vi "Generate Table.vi"() -> ()   [LabVIEW 2017]
panel:
  in  "Distance of Sensor Front to Back":dbl=34.0
  out "min time (in/sec)":dbl
  out "Feet/sec":dbl
  out "Distance":dbl
  out "Angle":dbl
  in  "Tape Width":dbl=2.0
  in  "Distance of Sensors Left to Right":dbl=20.0
  in  "Time between Rise of one to fall of other":dbl
  in  "Velocity(in/s":dbl=200.0
  out "Waveform Graph":waveform(dbl)(graph)
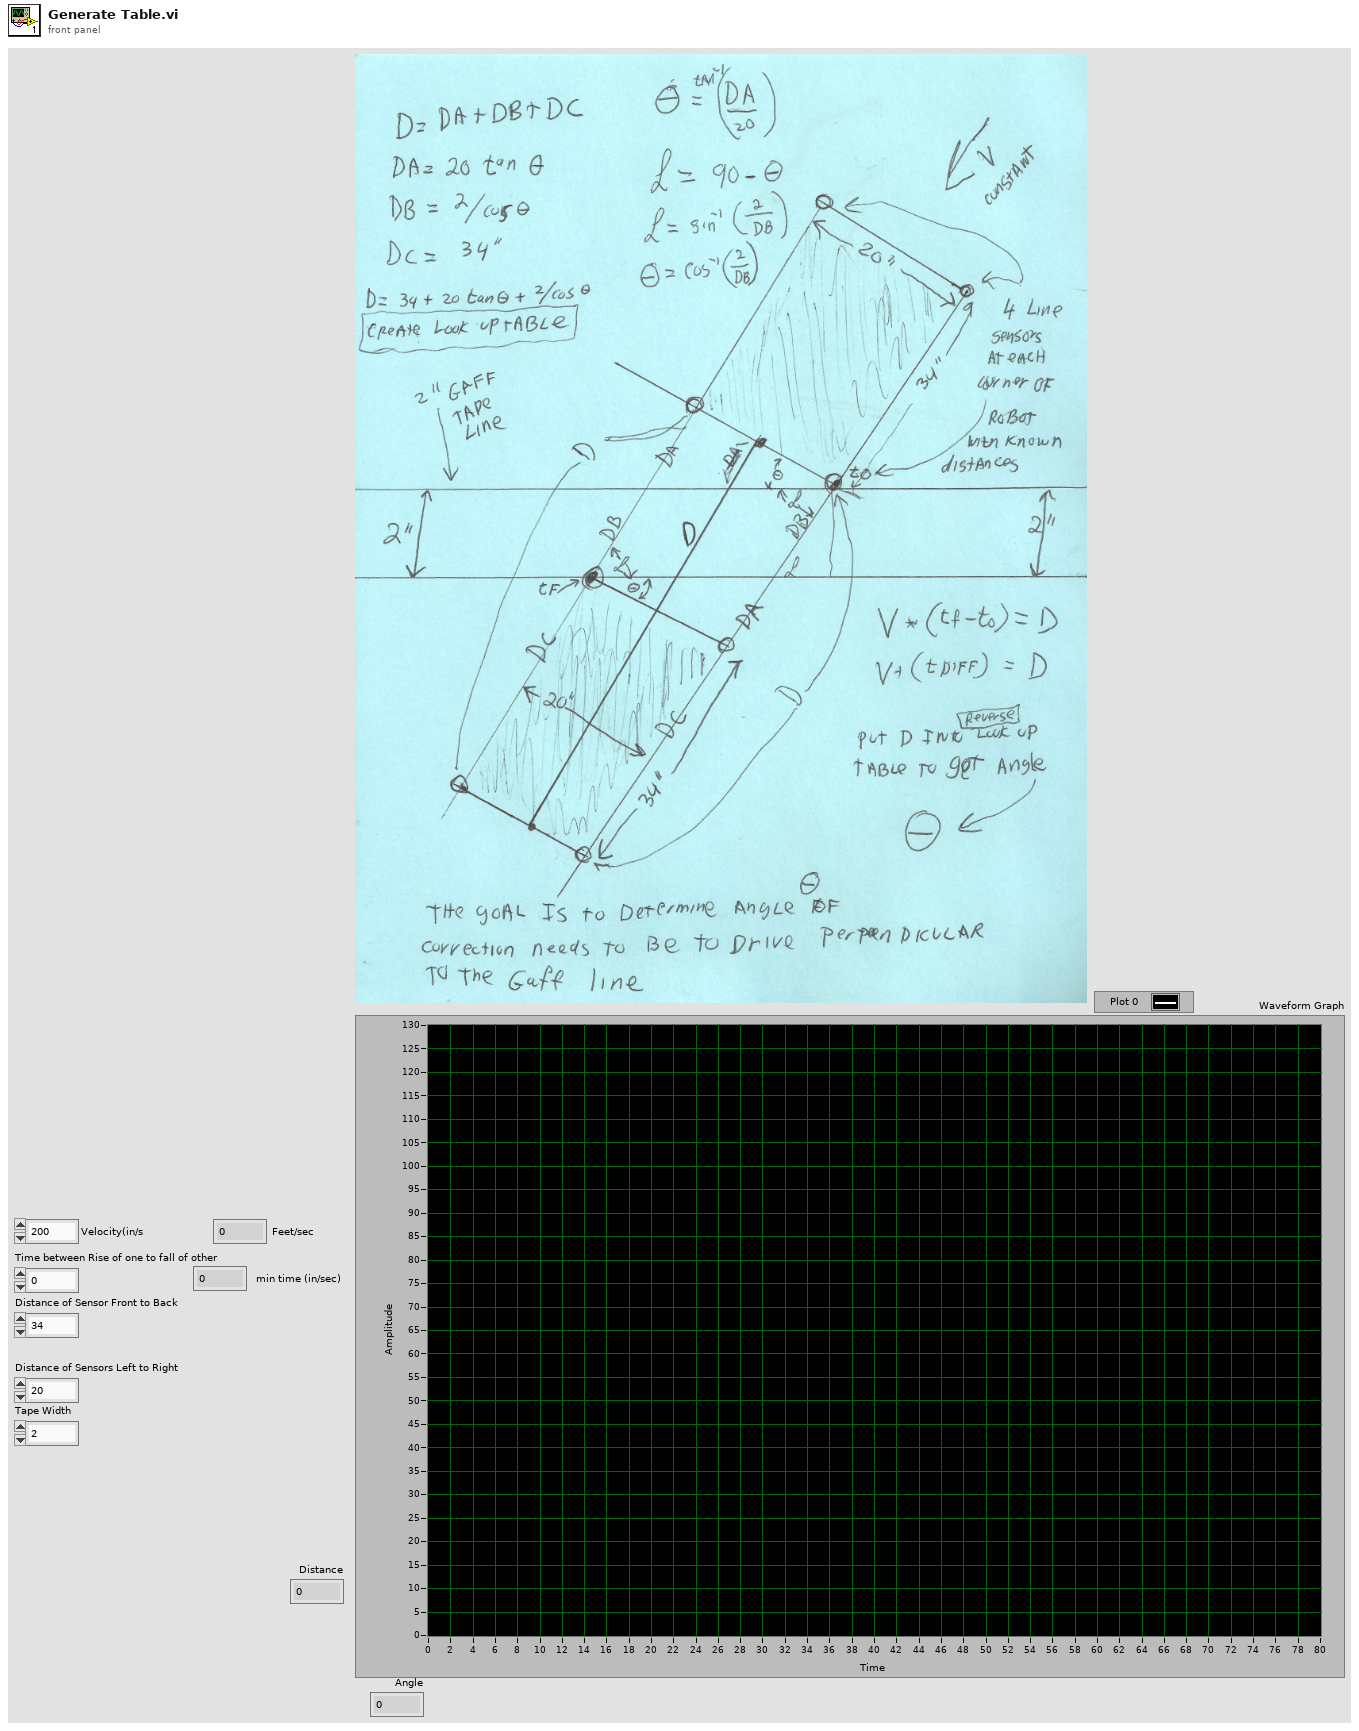
[diagram p1: front panel]
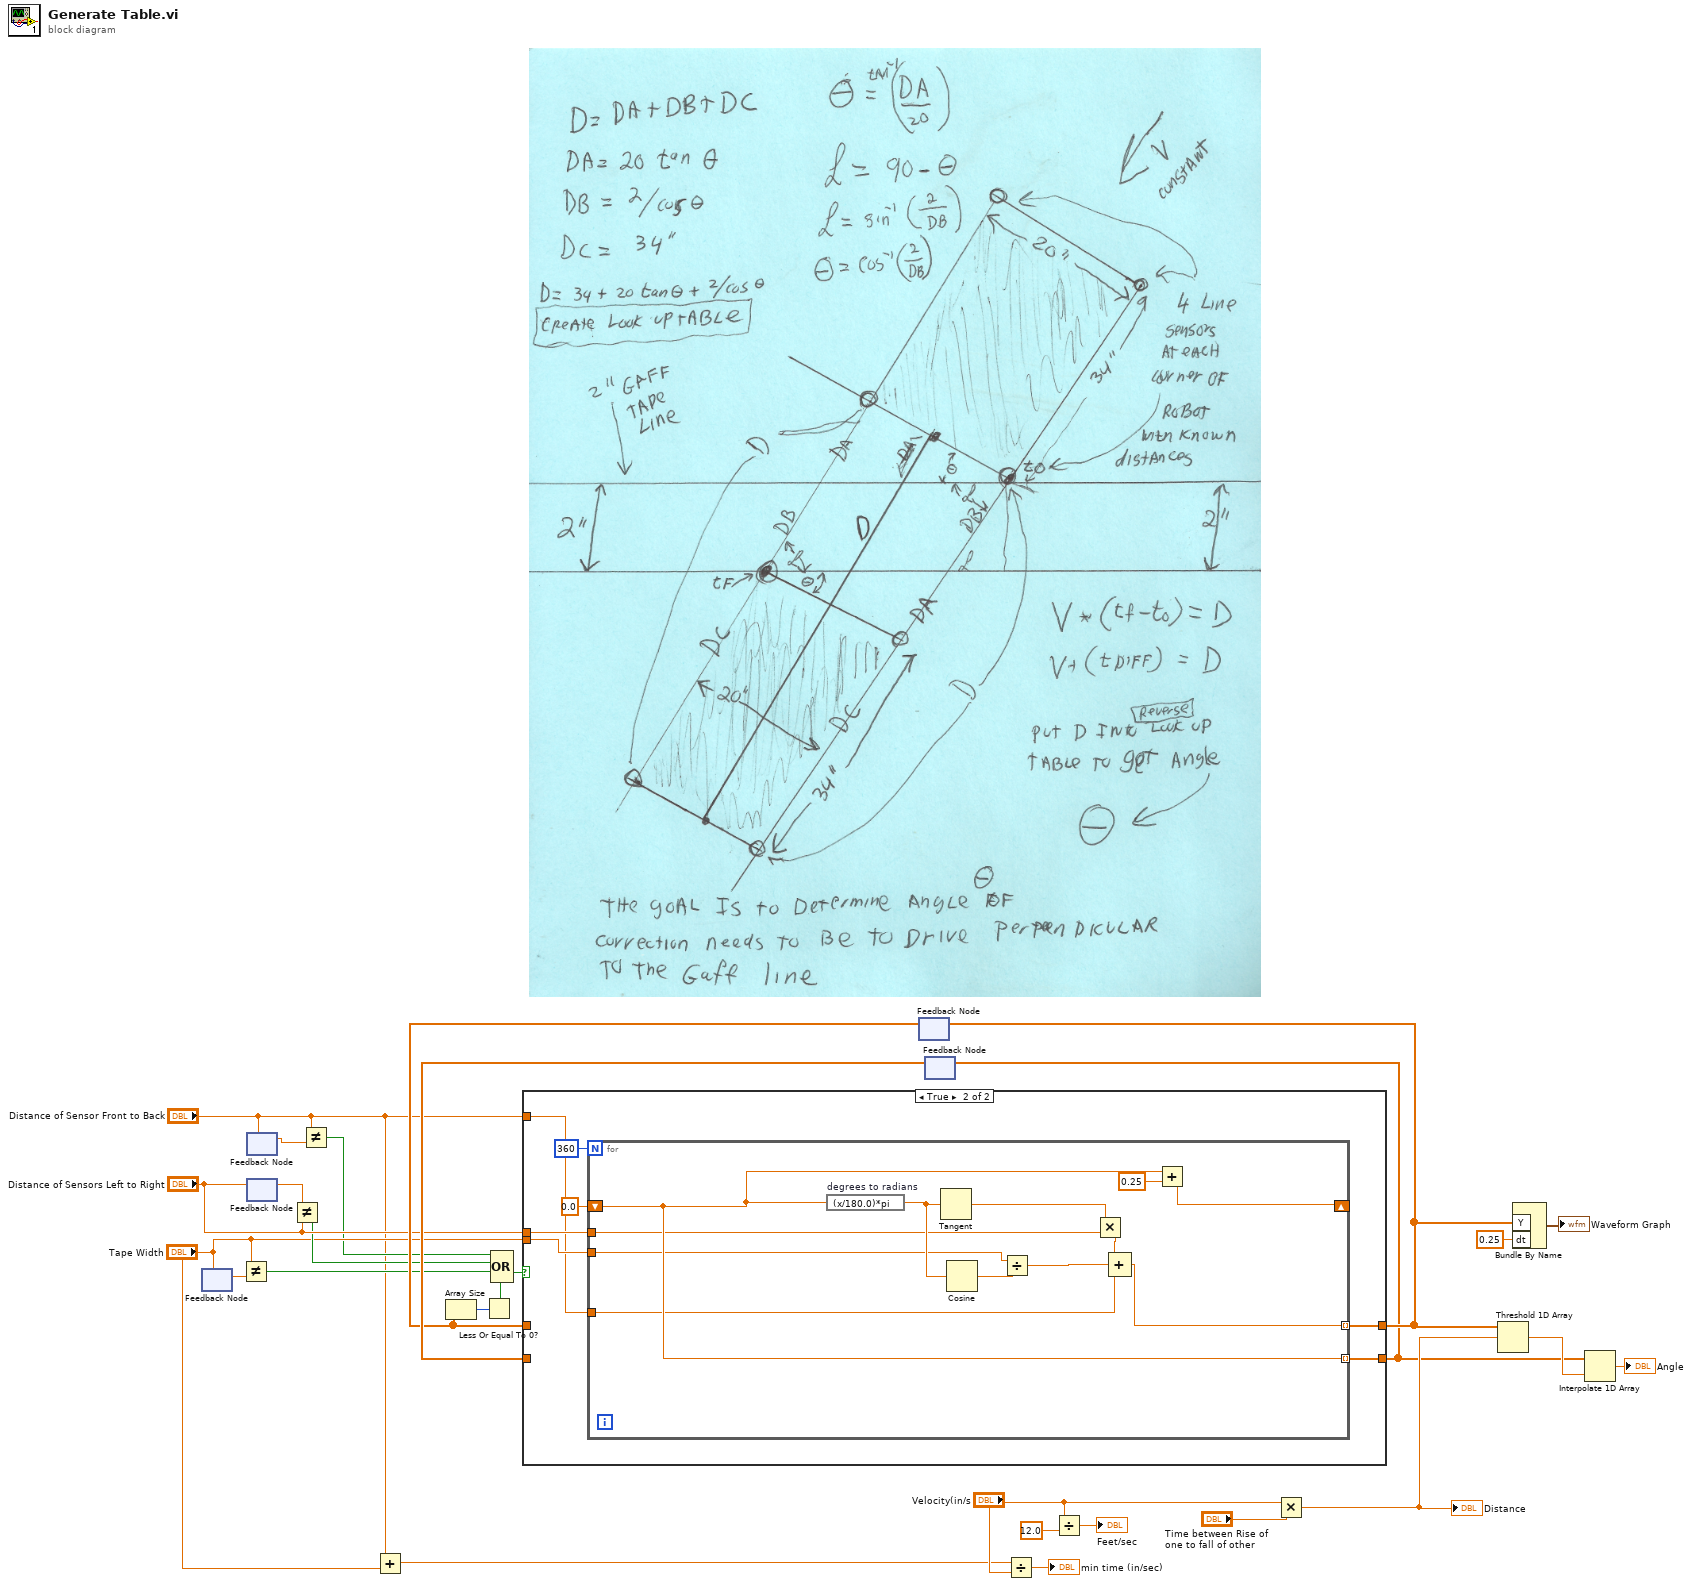
[diagram p0: block diagram]
diagram:
  n1 = feedback-in #1("Tape Width") -> ()
  n2 = feedback #1() -> (w14:dbl)  [unwired: 1 in]
  n3 = Not Equal?(x="Tape Width", y=w14) -> (x != y?=w13:bool)
  n4 = feedback #2() -> (w4:dbl)  [unwired: 1 in]
  n5 = feedback-in #2("Distance of Sensor Front to Back") -> ()
  n6 = feedback #3() -> (w11:dbl)  [unwired: 1 in]
  n7 = feedback-in #3("Distance of Sensors Left to Right") -> ()
  n8 = Not Equal?(x=w11, y="Distance of Sensors Left to Right") -> (x != y?=w10:bool)
  n9 = Not Equal?(x="Distance of Sensor Front to Back", y=w4) -> (x != y?=w3:bool)
  n10 = Add(x="Distance of Sensor Front to Back", y="Tape Width") -> (x+y=w2:dbl)
  n11 = feedback #4() -> (w18:dbl[])  [unwired: 1 in]
  n12 = Array Size(array=w18) -> (size(s)=w17:i32)
  n13 = Less Or Equal To 0?(x=w17) -> (x <= 0?=w16:bool)
  n14 = Compound Arithmetic op=OR(w3, w10, w13, w16) -> (w15:bool)
  n15 = feedback #5() -> (w19:dbl[])  [unwired: 1 in]
  n16 = case shown="True" w15 {
    tunnel: [w29 w35] -> w21
    tunnel: [w28 w34] -> w20
    tunnel: w18 -> [w29 _]
    tunnel: w19 -> [w28 _]
    tunnel: "Tape Width" -> [_ w33]
    tunnel: "Distance of Sensors Left to Right" -> [_ w32]
    tunnel: "Distance of Sensor Front to Back" -> [_ w30]
    frame False {
    }
    frame True {
      n17 = for {
        N: 360 -> [_]
        shift-right: [w43] -> _
        shift-left: 0.0 -> [w40]
        tunnel: [w42] -> w35 mode=indexing
        tunnel: [w40] -> w34 mode=indexing
        tunnel: w33 -> [w39]
        tunnel: w32 -> [w38]
        tunnel: w30 -> [w37]
        n18 = expression code="(x/180.0)*pi" "degrees to radians"(w40) -> (w41:dbl)
        n19 = Tangent(1:w41) -> (0:w48:dbl)
        n20 = Cosine(x=w41) -> (cos(x)=w47:dbl)
        n21 = Divide(x=w39, y=w47) -> (x/y=w45:dbl)
        n22 = Multiply(x=w48, y=w38) -> (x*y=w46:dbl)
        n23 = Compound Arithmetic op=ADD(w46, w45, w37) -> (w42:dbl)
        n24 = Add(x=w40, y=0.25) -> (x+y=w43:dbl)
      }
    }
  }
  n25 = feedback-in #4(w21) -> ()
  n26 = feedback-in #5(w20) -> ()
  n27 = Divide(x=w2, y="Velocity(in/s") -> (x/y=→"min time (in/sec)":dbl)
  n28 = Divide(x="Velocity(in/s", y=12.0) -> (x/y=→"Feet/sec":dbl)
  n29 = Multiply(x="Velocity(in/s", y="Time between Rise of one to fall of other") -> (x*y=w22:dbl)
  "Distance" <- w22
  n30 = Threshold 1D Array(2:w22, 3:w21) -> (0:w25:dbl)  [unwired: 1 in]
  n31 = Bundle By Name("Y"=w21, "dt"=0.25) -> (→"Waveform Graph":waveform(dbl))  [unwired: 1 in]
  n32 = Interpolate 1D Array(1:w25, 2:w20) -> (0:→"Angle":dbl)
